vi "Msg Remain.vi"(10 "Remaining Elements":refnum<class "Msg.lvclass">[](array[class]), 11 "Msg Remain in":refnum<class "Msg Remain.lvclass">) -> ()   [LabVIEW 2021, in "LVCAM.lvlib" / "Msg Remain.lvclass"]
uses:
  Msg Remain.lvclass
  Msg/Msg.lvclass
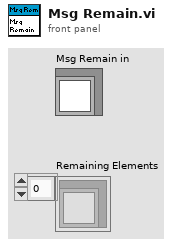
[diagram p1: front panel]
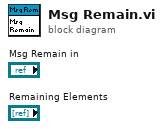
[diagram p0: block diagram]
diagram:
